vi "Write Data Entry Limits.vi"(8 "error in (no error)":errorcluster, 10 "Data Entry Limits":T1, 11 "Numeric.lvclass in":refnum<class "Numeric.lvclass">) -> (0 "error out":errorcluster, 3 "Numeric.lvclass out":refnum<class "Numeric.lvclass">)   [LabVIEW 2015, in "Numeric.lvclass"]
uses:
  Numeric.lvclass
  <vilib>/Utility/miscctls.llb/LVMinMaxIncTypeDef.ctl
  Numeric.lvclass/Numeric.ctl
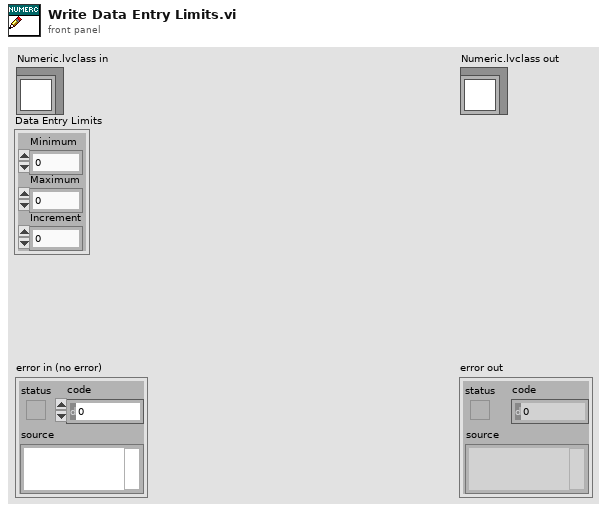
[diagram p1: front panel]
types:
  T1 = typedef "LVMinMaxIncTypeDef.ctl" = cluster{"Minimum":dbl, "Maximum":dbl, "Increment":dbl}
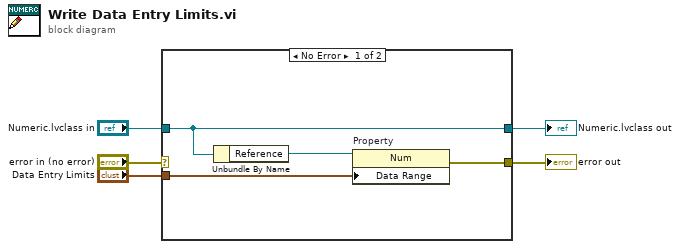
[diagram p0: block diagram]
diagram:
  n1 = case shown="No Error" "error in (no error)" {
    selector: "error in (no error)" -> [_ w11]
    tunnel: [w9 w11] -> w4
    tunnel: [w7 w10] -> w2
    tunnel: "Numeric.lvclass in" -> [w7 w10]
    tunnel: "Data Entry Limits" -> [w8 _]
    frame No Error {
      n2 = Unbundle By Name(w7) -> ("Reference"=w6:refnum<vi>)
      n3 = property on="Property" class="Num"(reference=w6, "Data Range"=w8) -> (error out=w9:errorcluster)  [unwired: 1 in, 1 out]
    }
    frame Error {
    }
  }
  "error out" <- w4
  "Numeric.lvclass out" <- w2
